vi "Get Panel Subpanel Refnum.vi"(8 "error in (no error)":errorcluster, 11 "Panel View in":refnum<class "Panel View.lvclass">) -> (0 "error out":errorcluster, 2 "Panel Subpanel Refnum":refnum<vi>, 3 "Panel View out":refnum<class "Panel View.lvclass">)   [LabVIEW 2015, in "Panel View.lvclass"]
uses:
  Panel View.lvclass
  Panel View.lvclass/Panel View.ctl
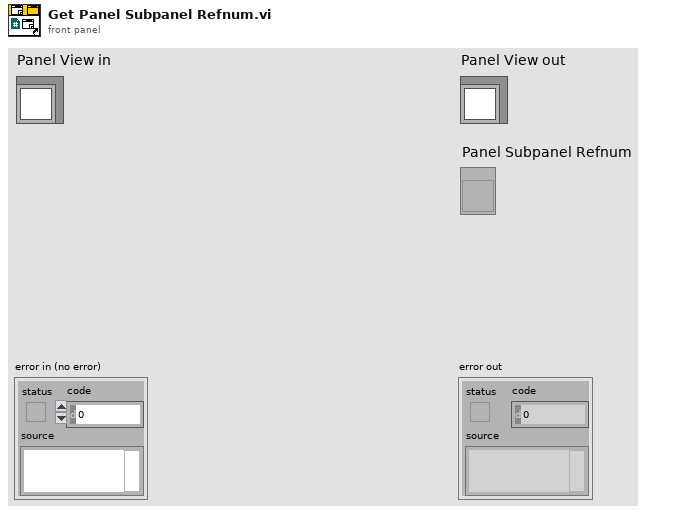
[diagram p1: front panel]
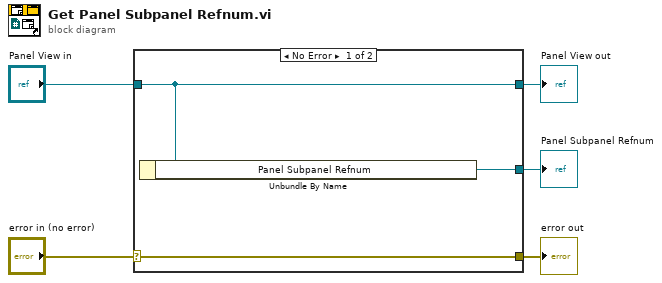
[diagram p0: block diagram]
diagram:
  n1 = case shown="No Error" "error in (no error)" {
    selector: "error in (no error)" -> [w8 w9]
    tunnel: [w8 w9] -> w4
    tunnel: [w7 w10] -> w2
    tunnel: "Panel View in" -> [w7 w10]
    tunnel: [w6 _] -> w1
    frame No Error {
      n2 = Unbundle By Name(w7) -> ("Panel Subpanel Refnum"=w6:refnum<vi>)
    }
    frame Error {
    }
  }
  "error out" <- w4
  "Panel View out" <- w2
  "Panel Subpanel Refnum" <- w1
